vi "Reception.vi"(0 "entrée d'erreur (pas d'erreur)":errorcluster, 1 "Nom de ressource VISA":refnum<visa-resource-name>) -> (2 "Sortie d'erreur":errorcluster caption="entrée d'erreur (pas d'erreur)", 3 "Checksum OK?":bool=TRUE, 4 "Data":dbl format="%.2f", 5 "ID byte":i32)   [LabVIEW 2010]
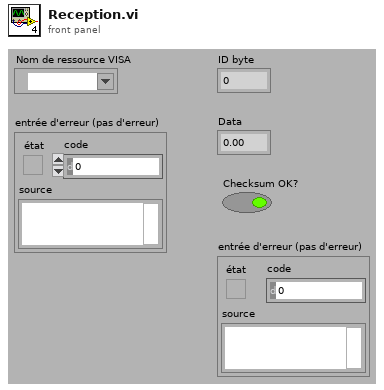
[diagram p1: front panel]
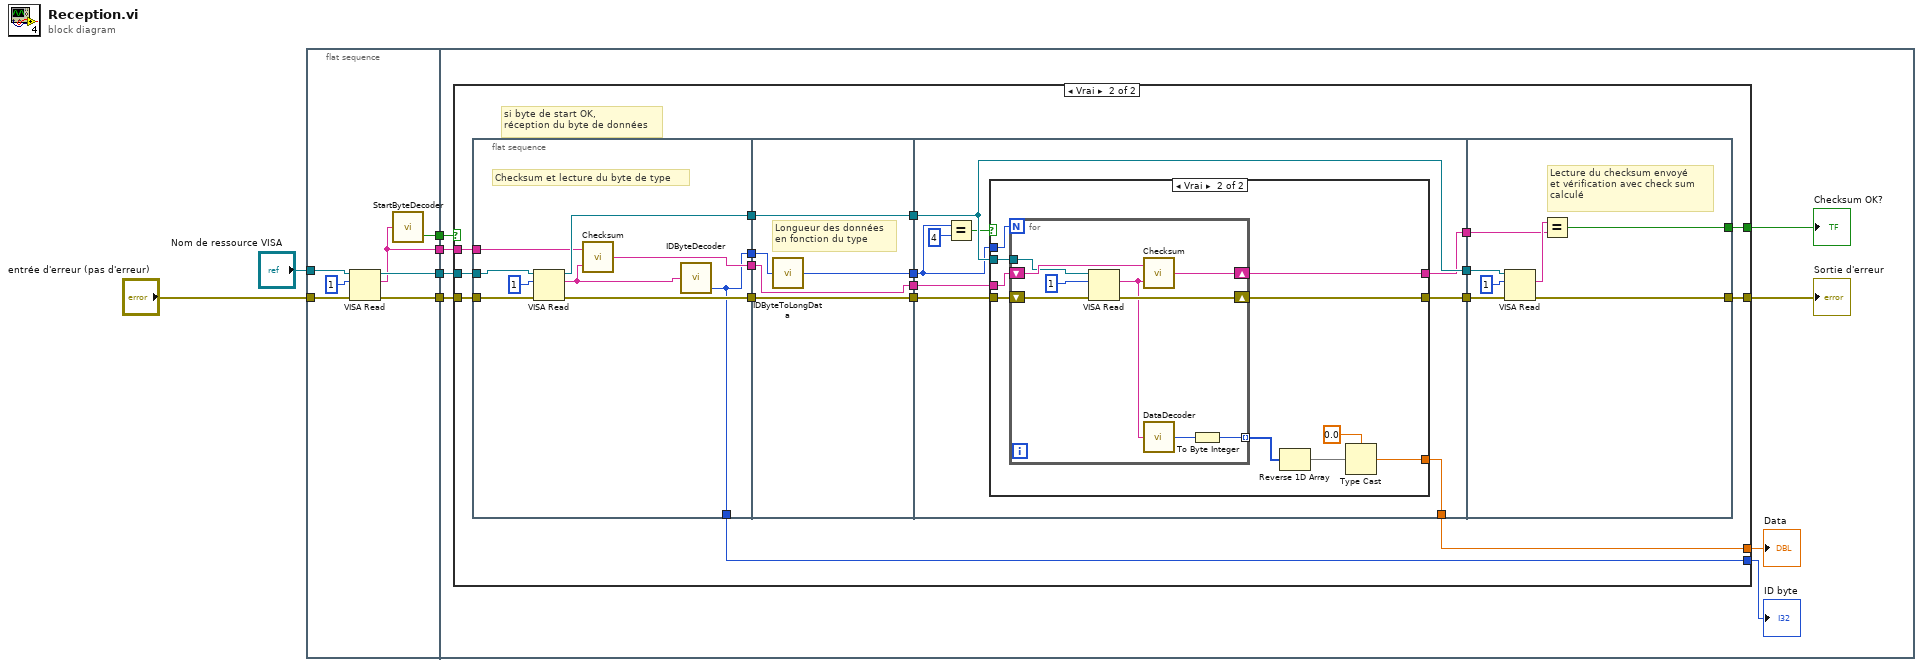
[diagram p0: block diagram]
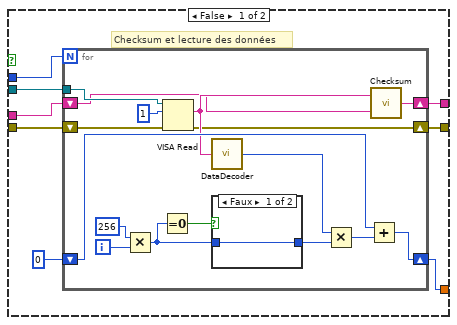
[diagram p3: hidden frame]
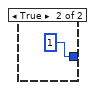
[diagram p4: hidden frame]
diagram:
  n1 = flat-sequence {
    tunnel: "Nom de ressource VISA" -> [w13]
    tunnel: "entrée d'erreur (pas d'erreur)" -> [w11]
    tunnel: [w10] -> w6
    tunnel: [w9] -> w5
    tunnel: [w8] -> w4
    tunnel: [w7] -> w3
    tunnel: w6 -> [w21]
    tunnel: w5 -> [w20]
    tunnel: w4 -> [w19]
    tunnel: w3 -> [w18]
    frame #0 {
      n2 = VISA Read(VISA resource name=w13, byte count=u32 1 ("nombre d'octets"), error in (no error)=w11) -> (VISA resource name out=w9:refnum<visa-resource-name>, read buffer=w7:string, error out=w8:errorcluster)  [unwired: 1 out]
      n3 = call "StartByteDecoder.vi"("byte1"=w7) -> ("Byte Start ?"=w10:bool)  [unwired: 1 in]
    }
    frame #1 {
      n4 = case shown="Vrai" w21 {
        tunnel: w20 -> [_ w40]
        tunnel: w19 -> [w22 w39]
        tunnel: w18 -> [_ w32]
        tunnel: [_ w26] -> w17
        tunnel: [_ w25] -> w16
        tunnel: [_ w24] -> w15
        tunnel: [w22 w23] -> w14
        frame False {
        }
        frame True {
          # "si byte de start OK,\nréception du byte de données"
          n5 = flat-sequence {
            tunnel: w40 -> [w49]
            tunnel: w39 -> [w47]
            tunnel: [w41] -> w38
            tunnel: [w46] -> w36
            tunnel: [w45] -> w34
            tunnel: w32 -> [w43]
            tunnel: [w42] -> w30
            tunnel: [w41] -> w26
            tunnel: w38 -> [w54]
            tunnel: [w53] -> w37
            tunnel: w36 -> [w52]
            tunnel: [w52] -> w35
            tunnel: w34 -> [w51]
            tunnel: [w51] -> w33
            tunnel: [w50] -> w31
            tunnel: w30 -> [w50]
            tunnel: w37 -> [w57]
            tunnel: w35 -> [w61]
            tunnel: w33 -> [w63]
            tunnel: w31 -> [w62]
            tunnel: [w61] -> w29
            tunnel: [w60] -> w28
            tunnel: [w59] -> w27
            tunnel: [w58] -> w25
            tunnel: w29 -> [w114]
            tunnel: w28 -> [w113]
            tunnel: w27 -> [w111]
            tunnel: [w110] -> w24
            tunnel: [w109] -> w23
            frame #0 {
              # "Checksum et lecture du byte de type"
              n6 = VISA Read(VISA resource name=w49, byte count=u32 1 ("nombre d'octets"), error in (no error)=w47) -> (VISA resource name out=w46:refnum<visa-resource-name>, read buffer=w44:string, error out=w45:errorcluster)  [unwired: 1 out]
              n7 = call "Checksum.vi"("Byte2"=w44, "Byte1"=w43) -> ("chaîne"=w42:string)
              n8 = call "IDByteDecoder.vi"("byte1"=w44) -> ("Type de donnee (ID)"=w41:i32)  [unwired: 2 out]
            }
            frame #1 {
              # "Longueur des données\nen fonction du type"
              n9 = call "IDByteToLongData.vi"("ID Byte"=w54) -> ("Data Long"=w53:i32)
            }
            frame #2 {
              n10 = Equal?(x=w57, y=4) -> (x = y?=w55:bool)
              n11 = case shown="Vrai" w55 {
                tunnel: w63 -> [w71 w95]
                tunnel: w57 -> [w70 w99]
                tunnel: w62 -> [w68 w98]
                tunnel: w61 -> [w67 w97]
                tunnel: [w66 w94] -> w60
                tunnel: [w65 w96] -> w59
                tunnel: [w64 w91] -> w58
                frame False {
                  # "Checksum et lecture des données"
                  n12 = for {
                    N: w70 -> [_]
                    tunnel: w67 -> [w87]
                    shift-right: [w79] -> w64
                    shift-left: 0 -> [w80]
                    shift-right: [w76] -> w65
                    shift-left: w68 -> [w77]
                    shift-right: [w75] -> w66
                    shift-left: w71 -> [w86]
                    i -> [w84]
                    n13 = Multiply(x=256, y=w84) -> (x*y=w72:i32)
                    n14 = Equal To 0?(x=w72) -> (x = 0?=w74:bool)
                    n15 = VISA Read(VISA resource name=w87, byte count=u32 1 ("nombre d'octets"), error in (no error)=w86) -> (read buffer=w78:string, error out=w75:errorcluster)  [unwired: 2 out]
                    n16 = call "DataDecoder.vi"("byte1"=w78) -> ("Data"=w82:i32)
                    n17 = case shown="Faux" w74 {
                      tunnel: [w88 1 ("x")] -> w73
                      tunnel: w72 -> [w88 _]
                      frame False {
                      }
                      frame True {
                      }
                    }
                    n18 = Multiply(x=w82, y=w73) -> (x*y=w81:i32)
                    n19 = Add(x=w80, y=w81) -> (x+y=w79:i32)
                    n20 = call "Checksum.vi"("Byte2"=w77, "Byte1"=w78) -> ("chaîne"=w76:string)
                  }
                }
                frame True {
                  n21 = for {
                    N: w99 -> [_]
                    shift-right: [w108] -> w96
                    shift-left: w98 -> [w107]
                    tunnel: w97 -> [w106]
                    shift-right: [w103] -> w94
                    shift-left: w95 -> [w104]
                    tunnel: [w100] -> w93 mode=indexing
                    n22 = VISA Read(VISA resource name=w106, byte count=u32 1 ("nombre d'octets"), error in (no error)=w104) -> (read buffer=w102:string, error out=w103:errorcluster)  [unwired: 2 out]
                    n23 = call "Checksum.vi"("Byte2"=w102, "Byte1"=w107) -> ("chaîne"=w108:string)
                    n24 = call "DataDecoder.vi"("byte1"=w102) -> ("Data"=w101:i32)
                    n25 = To Byte Integer(number=w101) -> (8bit integer=w100:i8)
                  }
                  n26 = Reverse 1D Array(array=w93) -> (reversed array=w90:i8[])
                  n27 = Type Cast(type=0.0, x=w90) -> (*(type *) &x=w91:dbl)
                }
              }
            }
            frame #3 {
              # "Lecture du checksum envoyé\net vérification avec check sum \ncalculé"
              n28 = VISA Read(VISA resource name=w114, byte count=u32 1 ("nombre d'octets"), error in (no error)=w113) -> (read buffer=w112:string, error out=w109:errorcluster)  [unwired: 2 out]
              n29 = Equal?(x=w112, y=w111) -> (x = y?=w110:bool)
            }
          }
        }
      }
      "ID byte" <- w17
      "Data" <- w16
      "Checksum OK?" <- w15
      "Sortie d'erreur" <- w14
    }
  }
